vi "Get Discovery Service Address.vi"(8 "error in":errorcluster, 11 "cluster id":string) -> (0 "error out":errorcluster, 3 "address":string)   [LabVIEW 2020, in "Measurement Plugin Measurement Server.lvlib"]
doc: "This VI is deprecated. Please use <b>MeasurementLink Discovery::Get Discovery Service Address.vi</b> for the same functionality."
uses:
  Measurement Plugin Measurement Server.lvlib
  Measurement Plugin Discovery V1/Measurement Plugin Discovery V1.lvlib
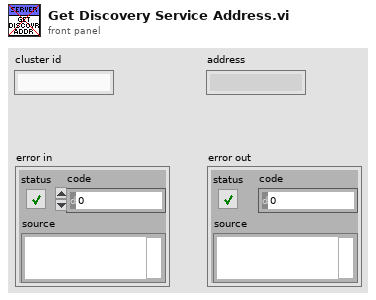
[diagram p1: front panel]
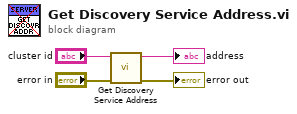
[diagram p0: block diagram]
diagram:
  n1 = call "Get Discovery Service Address.vi"("error in"="error in", "cluster id (\"\")"="cluster id") -> ("error out"=→"error out":errorcluster, "address"=→"address":string)  [unwired: 8 in]
